vi "VI esame mod.vi"() -> ()   [LabVIEW 2012]
uses:
  <vilib>/Analysis/baseanly.llb/Mean (DBL).vi
  <vilib>/Analysis/NI_AALBase.lvlib
panel:
  out "mean":dbl format="%0.2f"
  out "Waveform Graph":dbl[][](graph)
  out "output cluster":cluster{dbl[], dbl[], u32[]}
  out "vet max":u32[](array[numeric])
  out "output array":u32[](array[numeric])
  out "B N*15":u32[][](array[numeric])
  out "Array tempi":u32[](array[numeric])
  out "x+y":u32
  out "nuova matrice":dbl[][](array[numeric])
  out "vet smooting 3 elem":dbl[](array[numeric])
  out "result":dbl
  in  "n":i32
  out "n-esima riga":dbl[](array[numeric])
  out "subarray":dbl[][](array[numeric])
  out "A N*15":dbl[][](array[numeric])
  out "Array n":dbl[](array[numeric])
  out "number":dbl
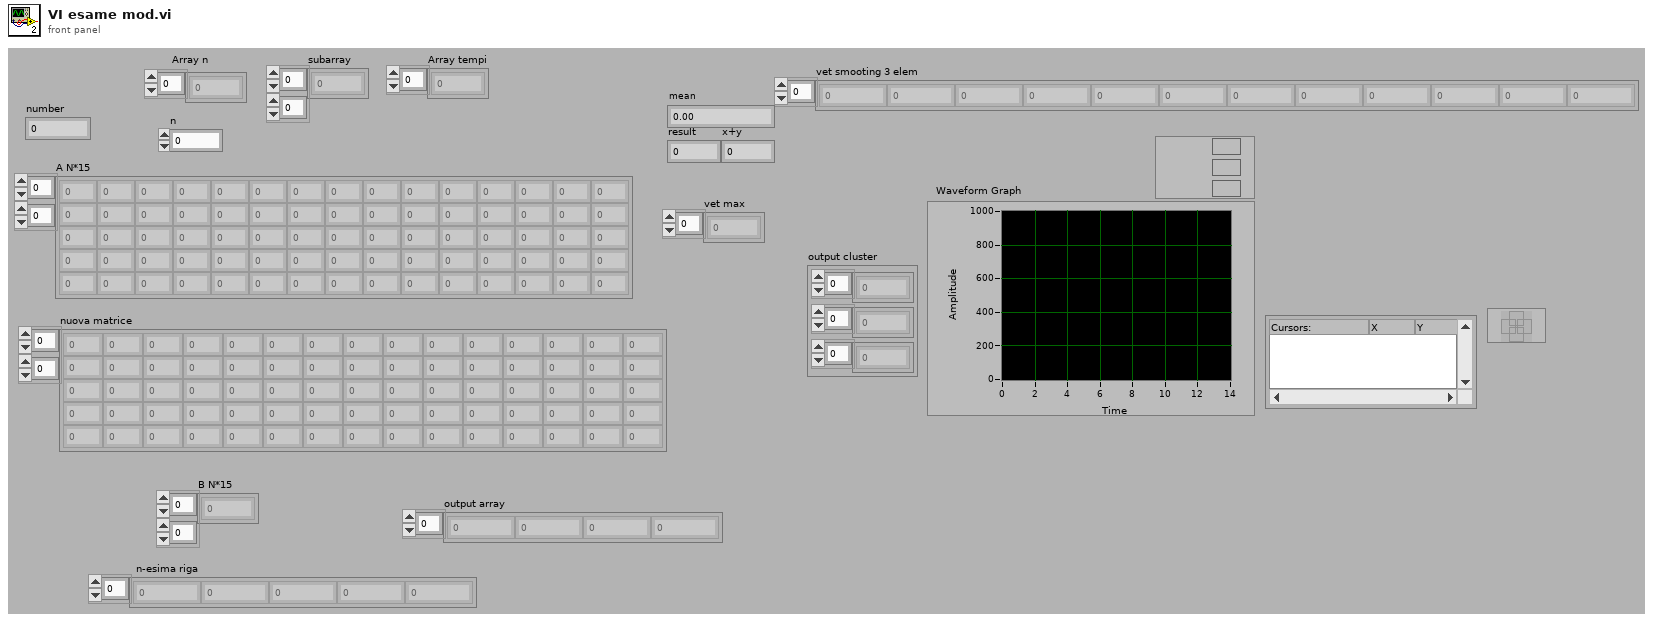
[diagram p1: front panel]
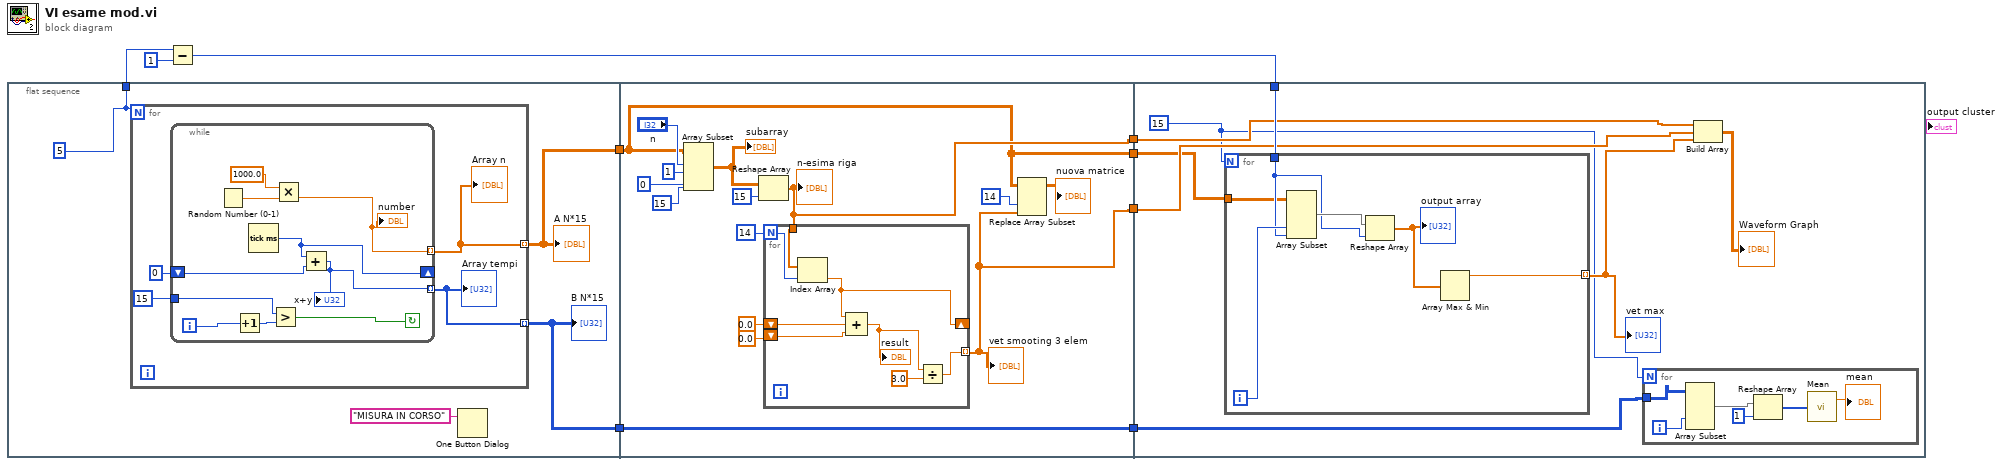
[diagram p0: block diagram]
diagram:
  n1 = flat-sequence {
    tunnel: [w13] -> w9
    tunnel: [w10] -> w6
    tunnel: [w11] -> w1
    tunnel: w9 -> [w30]
    tunnel: [w32] -> w8
    tunnel: [w31] -> w7
    tunnel: [w30] -> w3
    tunnel: [w29] -> w2
    tunnel: w1 -> [w29]
    tunnel: w8 -> [w57]
    tunnel: w7 -> [w56]
    tunnel: w4 -> [w58]
    tunnel: w3 -> [w53]
    tunnel: w2 -> [w52]
    frame #0 {
      w10 = 5
      n2 = for {
        N: w10 -> [_]
        tunnel: [w16] -> w13 mode=indexing
        tunnel: [w14] -> w11 mode=indexing
        n3 = while {
          tunnel: 15 -> [w25]
          tunnel: [w19] -> w16 mode=indexing
          shift-right: [w22] -> _
          shift-left: u32 0 -> [w23]
          tunnel: [w21] -> w14 mode=indexing
          i -> [w27]
          stop <- w24 continue-if-true
          n4 = Random Number (0-1)() -> (number: 0 to 1=w20:dbl)
          n5 = Increment(x=w27) -> (x+1=w26:i32)
          n6 = Tick Count (ms)() -> (millisecond timer value=w22:u32)
          n7 = Greater?(x=w25, y=w26) -> (0:w24:bool)
          n8 = Multiply(x=1000.0, y=w20) -> (x*y=w19:dbl)
          "number" <- w19
          n9 = Add(x=w22, y=w23) -> (x+y=w21:u32)
          "x+y" <- w21
        }
        "Array n" <- w16
        "Array tempi" <- w14
      }
      "A N*15" <- w13
      "B N*15" <- w11
      n10 = One Button Dialog(message="MISURA IN CORSO") -> ()  [unwired: 1 in, 1 out]
    }
    frame #1 {
      n11 = Array Subset(array=w30, index (row)="n", length (row)=1 ("length"), index (col)=0 ("index"), length (col)=15 ("length")) -> (w39:dbl[][])
      "subarray" <- w39
      n12 = Reshape Array(w39, 15 ("dimension size")) -> (w32:dbl[])
      "n-esima riga" <- w32
      n13 = for {
        N: 14 -> [w43]
        tunnel: w32 -> [w50]
        shift-right: [w44] -> _
        shift-left: 0.0 -> [w49]
        shift-left: 0.0 -> [w48]
        tunnel: [w45] -> w31 mode=indexing
        n14 = Index Array(array=w50, index=w43) -> (element=w44:dbl)
        n15 = Compound Arithmetic op=ADD(w44, w49, w48) -> (w46:dbl)
        "result" <- w46
        n16 = Divide(x=w46, y=3.0) -> (x/y=w45:dbl)
      }
      "vet smooting 3 elem" <- w31
      n17 = Replace Array Subset(array=w30, new element=w31, index (col)=14 ("index (row)")) -> (→"nuova matrice":dbl[][])  [unwired: 1 in]
    }
    frame #2 {
      w51 = 15
      n18 = for {
        N: w51 -> [_]
        tunnel: w58 -> [w68]
        tunnel: [w66] -> w55 mode=indexing
        tunnel: w53 -> [w65]
        i -> [w70]
        n19 = Array Subset(array=w65, index (col)=w70, length (col)=w68) -> (w69:dbl[][])  [unwired: 2 in]
        n20 = Reshape Array(w69, w68) -> (w67:dbl[])
        "output array" <- w67
        n21 = Array Max & Min(array=w67) -> (max value=w66:dbl)  [unwired: 3 out]
      }
      "vet max" <- w55
      n22 = for {
        N: w51 -> [_]
        tunnel: w52 -> [w64]
        i -> [w63]
        n23 = Array Subset(array=w64, index (col)=w63) -> (w62:u32[][])  [unwired: 3 in]
        n24 = Reshape Array(w62, 1 ("dimension size")) -> (w61:u32[])
        n25 = call-poly <vilib>:"Mean.vi"("X"=w61) -> ("mean"=→"mean":dbl)  [unwired: 1 out]
      }
      n26 = Build Array(w57, w56, w55) -> (→"Waveform Graph":dbl[][])
    }
  }
  n27 = Subtract(x=w6, y=1) -> (x-y=w4:i32)
